vi "Auto Further Switch.vi"(10 "Time to wait (min 50ms)":dbl=100.0, 11 "Right?":bool) -> ()   [LabVIEW 2017]
uses:
  LabVIEW_is_Under_Control.lib/Util/Unpack Gamepad/Button Cluster.ctl
  Team Code/Robot Global Data.vi
panel:
  out "Auto State":T1(ring)
  in  "Time_Limit_ Turn_2":dbl=1500.0 format="%#_13g"
  in  "Time_Limit_fwd_2":dbl=4000.0 format="%#_13g"
  in  "Time_Limit_Turn":dbl=1500.0 format="%#_13g"
  in  "Time_Limit_fwd":dbl=4000.0 format="%#_13g"
  in  "Time_Limit_fwd_3":dbl=1000.0 format="%#_13g"
  in  "Time to wait 3(min 50ms)":dbl=50.0
  in  "Delay Fwd 3":i32=500
  in  "Distance fwd 3":dbl=50.0
  in  "Delay Turn 2":i32=200
  in  "Turn 2":dbl=-90.0 format="%#_13g"
  in  "Delay Fwd 2":i32=200
  in  "Distance fwd 2":dbl=430.0
  in  "Delay Turn":i32=300
  in  "Turn":dbl=-90.0 format="%#_13g"
  in  "Delay Fwd":i32=600
  in  "Distance fwd 1":dbl=600.0
  in  "Time to wait 3 (min 50ms)":dbl=50.0
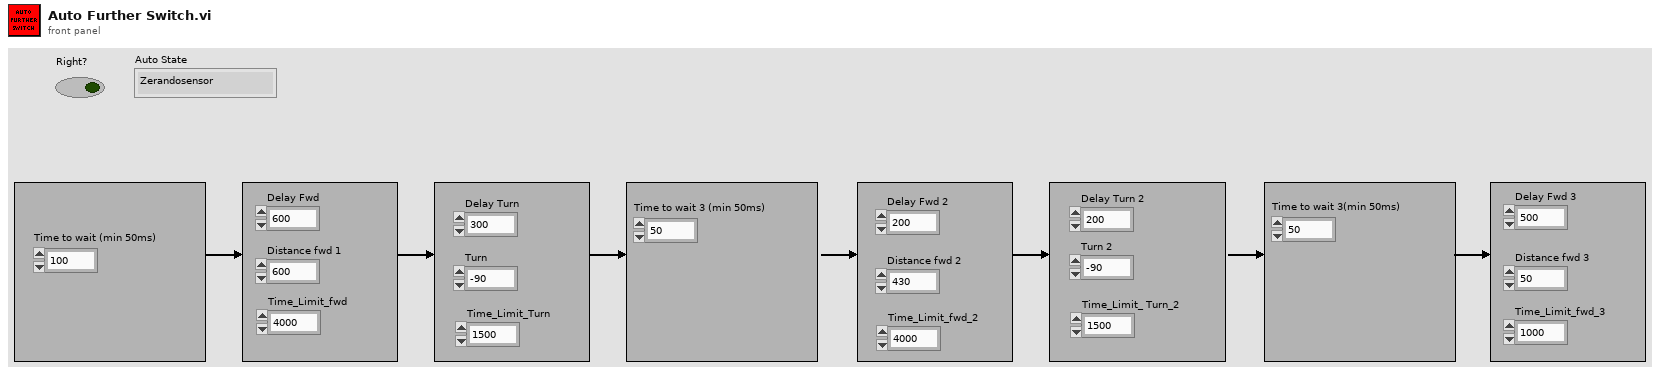
[diagram p1: front panel]
types:
  T1 = enum16{"Zerandosensor", "Andando", "Girando", "Zerandosensor2", "Andando2", "Girando2", "Zerandosensor3", "Andando3", "Score", "Finalizando", "Jogando"}
  T2 = enum16{"Zerandosensor", "Andando", "Girando", "Zerandosensor2", "Andando2", "Girando2", "Zerandosensor3", "Andando3", "Score", "Finalizando"}
  T3 = typedef "Button Cluster.ctl" = cluster{"Buttons[0]":bool, "Buttons[1]":bool, "Buttons[2]":bool, "Buttons[3]":bool, "Buttons[4]":bool, "Buttons[5]":bool, "Buttons[6]":bool, "Buttons[7]":bool, "Buttons[8]":bool, "Buttons[9]":bool}
  T4 = cluster{"proportional gain (Kc)":dbl, "integral time (Ti, min)":dbl, "derivative time (Td, min)":dbl}
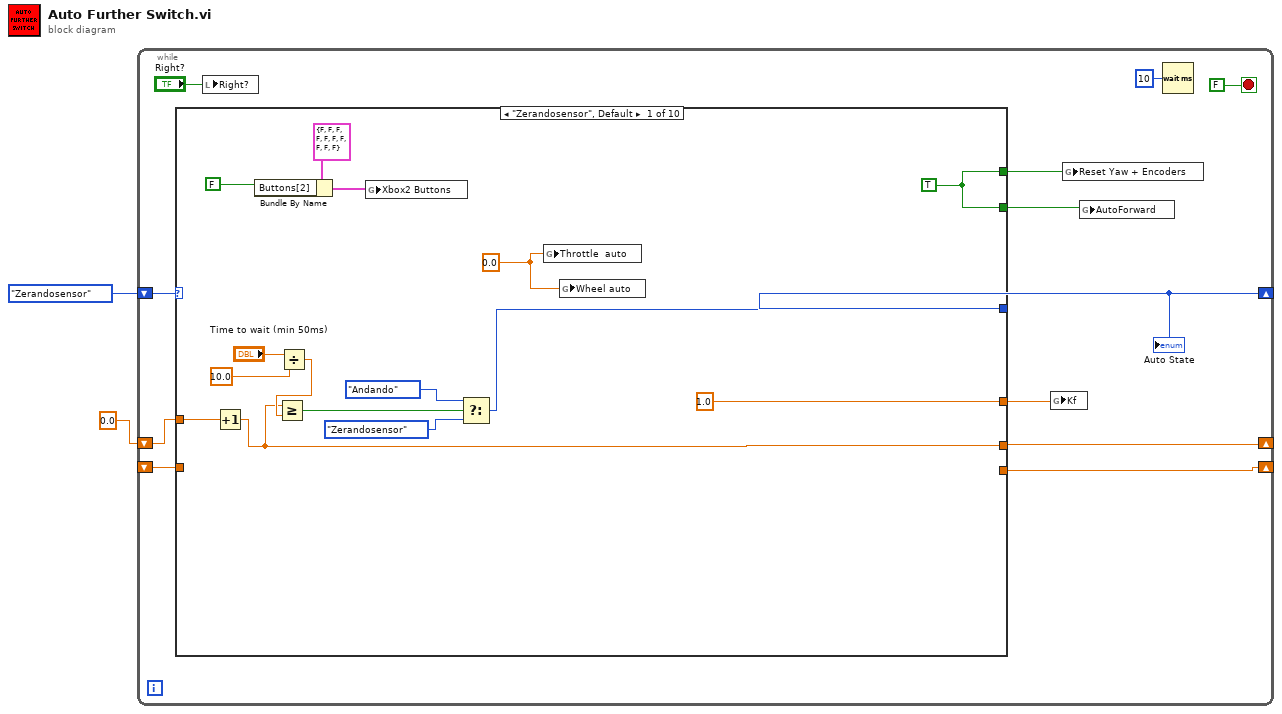
[diagram p0: block diagram]
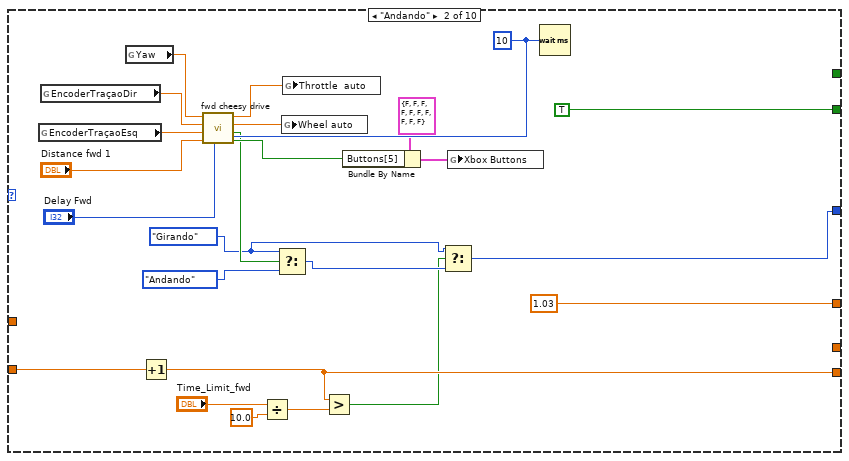
[diagram p2: hidden frame]
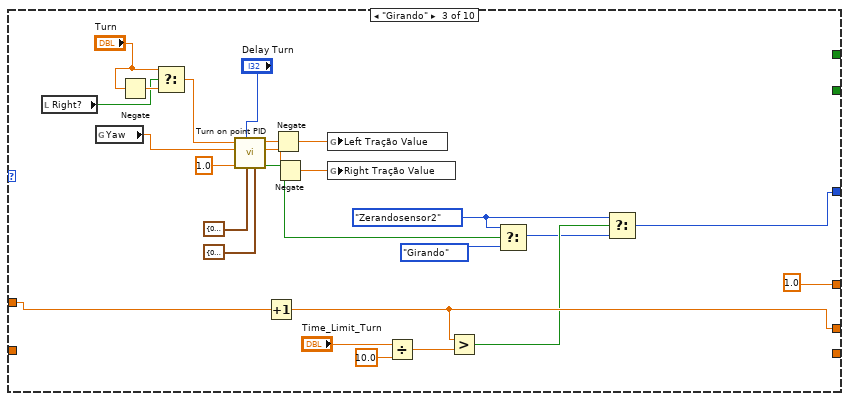
[diagram p3: hidden frame]
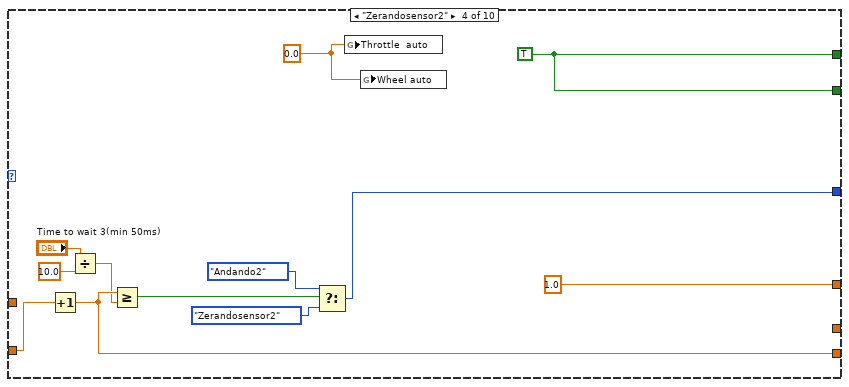
[diagram p4: hidden frame]
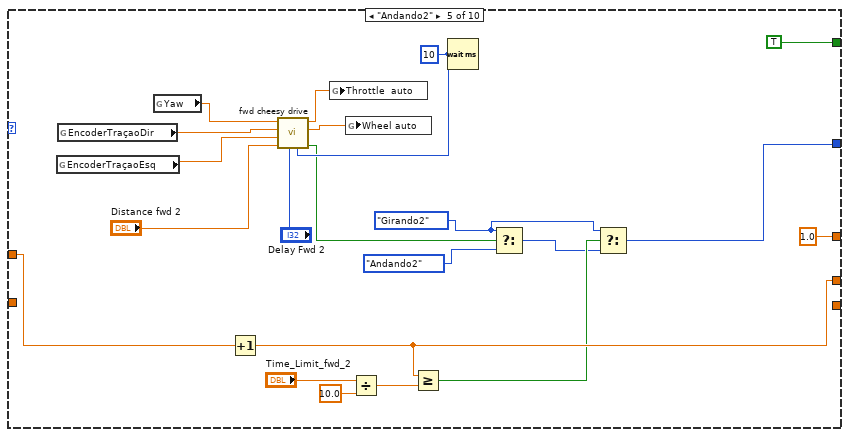
[diagram p5: hidden frame]
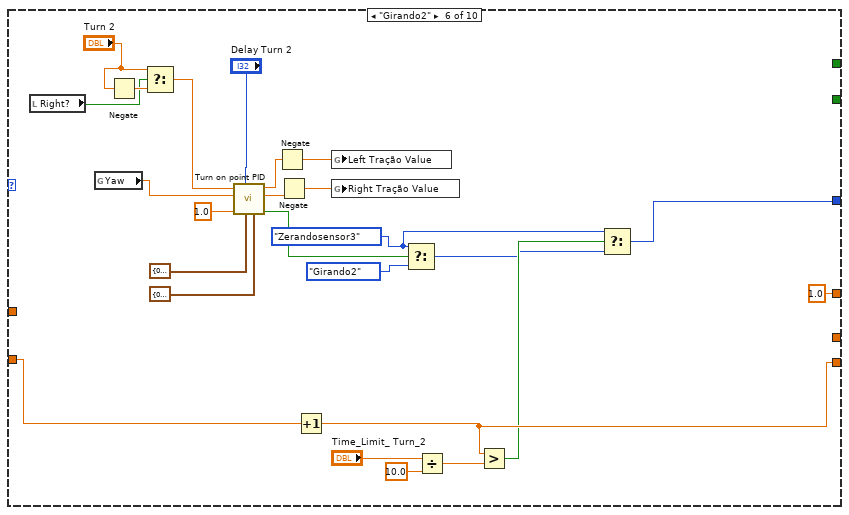
[diagram p6: hidden frame]
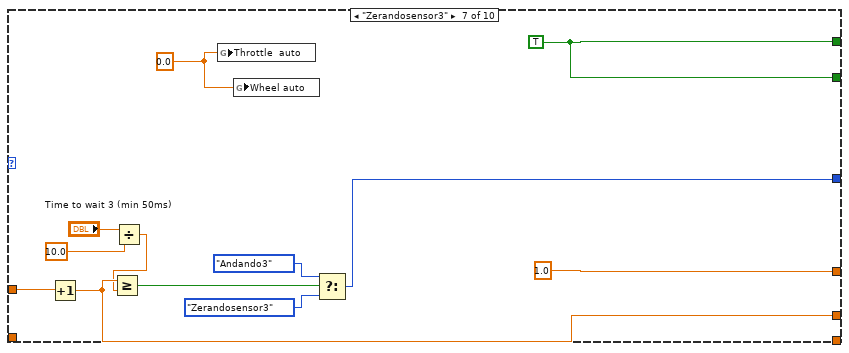
[diagram p7: hidden frame]
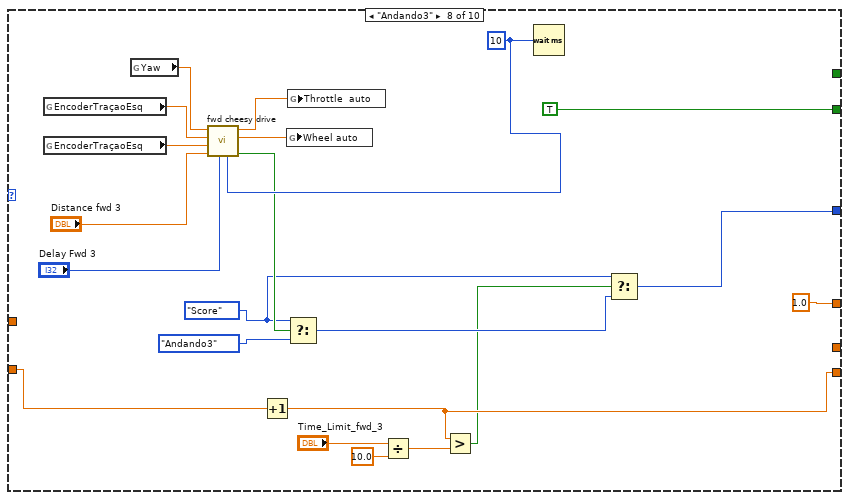
[diagram p8: hidden frame]
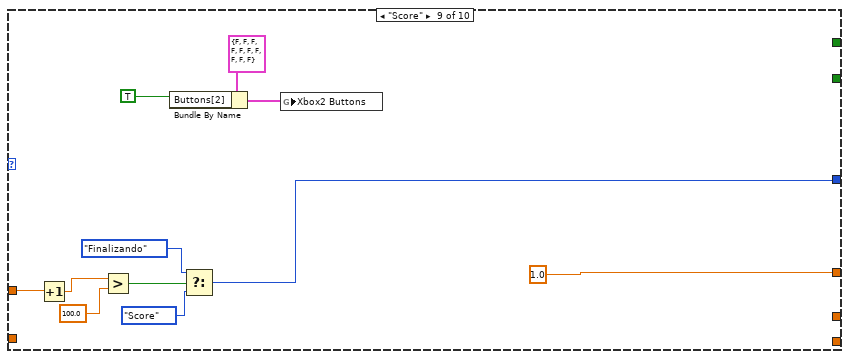
[diagram p9: hidden frame]
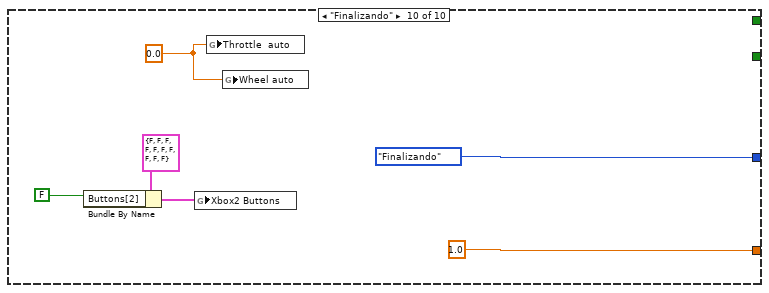
[diagram p10: hidden frame]
diagram:
  n1 = while {
    shift-right: [w6] -> _
    shift-left: T2."Zerandosensor" -> [w5]
    shift-right: [w8] -> _
    shift-left: 0.0 -> [w9]
    shift-right: [w3] -> _
    shift-left: _ -> [w4]
    stop <- FALSE stop-if-true
    n2 = case shown="\"Zerandosensor\", Default" w5 {
      tunnel: [w29 _ _ w88 _ _ w142 _ _ _] -> w11
      tunnel: [w29 TRUE _ w88 TRUE _ w142 TRUE _ _] -> w12
      tunnel: [1.0 1.03 1.0 1.0 1.0 1.0 1.0 1.0 1.0 1.0] -> w10
      tunnel: w9 -> [w25 _ w59 _ w96 _ w146 _ w180 _]
      tunnel: [w15 _ w58 _ w95 _ w138 _ _ _] -> w8
      tunnel: [w22 w34 w57 w86 w91 w116 w141 w153 w173 T1."Finalizando"] -> w6
      tunnel: w4 -> [_ w36 _ w83 _ w118 _ w155 _ _]
      tunnel: [_ w35 _ w82 _ w117 _ w154 _ _] -> w3
      frame "Zerandosensor", Default {
        w23 = 0.0
        w29 = TRUE
        n3 = Increment(x=w25) -> (x+1=w15:dbl)
        n4 = Bundle By Name(cluster=T3 {"Buttons[0]"=FALSE, "Buttons[1]"=FALSE, "Buttons[2]"=FALSE, "Buttons[3]"=FALSE, "Buttons[4]"=FALSE, "Buttons[5]"=FALSE, "Buttons[6]"=FALSE, "Buttons[7]"=FALSE, "Buttons[8]"=FALSE, "Buttons[9]"=FALSE} ("Xbox Buttons"), "Buttons[2]"=FALSE) -> (w18:T3)
        n5 = Divide(x="Time to wait (min 50ms)", y=10.0) -> (x/y=w16:dbl)
        n6 = Greater Or Equal?(x=w15, y=w16) -> (x >= y?=w24:bool)
        n7 = global write "Robot Global Data.vi" "Xbox2 Buttons"(w18) -> ()
        n8 = Select(t=T2."Andando", s=w24, f=T2."Zerandosensor") -> (s? t:f=w22:T2)
        n9 = global write "Robot Global Data.vi" "Throttle  auto"(w23) -> ()
        n10 = global write "Robot Global Data.vi" "Wheel auto"(w23) -> ()
      }
      frame "Andando" {
        w31 = T2."Girando"
        w47 = u32 10 ("milliseconds to wait")
        n11 = global read "Robot Global Data.vi" "EncoderTraçaoEsq"() -> (w50:dbl)
        n12 = global read "Robot Global Data.vi" "EncoderTraçaoDir"() -> (w49:dbl)
        n13 = global read "Robot Global Data.vi" "Yaw"() -> (w51:dbl)
        n14 = Increment(x=w36) -> (x+1=w35:dbl)
        n15 = call "fwd cheesy drive.vi"("Loop Timer"=w47, "Time to stop"="Delay Fwd", "Distance"="Distance fwd 1", "Encoder Left"=w50, "Encoder Right"=w49, "Yaw"=w51) -> ("Finished distance"=w42:bool, "Both finished"=w41:bool, "Direction"=w46:dbl, "Trottle"=w45:dbl)  [unwired: 2 in]
        n16 = Divide(x="Time_Limit_fwd", y=10.0) -> (x/y=w39:dbl)
        n17 = Select(t=w31, s=w41, f=T2."Andando") -> (s? t:f=w32:T2)
        n18 = global write "Robot Global Data.vi" "Wheel auto"(w46) -> ()
        n19 = global write "Robot Global Data.vi" "Throttle  auto"(w45) -> ()
        n20 = Greater?(x=w35, y=w39) -> (0:w30:bool)
        n21 = Bundle By Name(cluster=T3 {"Buttons[0]"=FALSE, "Buttons[1]"=FALSE, "Buttons[2]"=FALSE, "Buttons[3]"=FALSE, "Buttons[4]"=FALSE, "Buttons[5]"=FALSE, "Buttons[6]"=FALSE, "Buttons[7]"=FALSE, "Buttons[8]"=FALSE, "Buttons[9]"=FALSE} ("Xbox Buttons"), "Buttons[5]"=w42) -> (w43:T3)
        n22 = Select(t=w31, s=w30, f=w32) -> (s? t:f=w34:T2)
        n23 = global write "Robot Global Data.vi" "Xbox Buttons"(w43) -> ()
        n24 = Wait (ms)(milliseconds to wait=w47) -> ()  [unwired: 1 out]
      }
      frame "Girando" {
        w54 = T2."Zerandosensor2"
        n25 = local read "Right?"() -> (w66:bool)
        n26 = global read "Robot Global Data.vi" "Yaw"() -> (w72:dbl)
        n27 = Negate(x="Turn") -> (-x=w69:dbl)
        n28 = Select(t="Turn", s=w66, f=w69) -> (s? t:f=w67:dbl)
        n29 = call "Turn on point PID.vi"("Range"=cluster{"output high":dbl, "output low":dbl} {"output high"=0.65, "output low"=-0.65}, "Gains"=T4 {"proportional gain (Kc)"=0.015, "integral time (Ti, min)"=0.01, "derivative time (Td, min)"=0.0}, "Time to stop"="Delay Turn", "Precision"=1.0, "Yaw"=w72, "Setpoint(degrees)"=w67) -> ("Finished?"=w76:bool, "PWM right"=w73:dbl, "PWM left"=w74:dbl)  [unwired: 3 in]
        n30 = Increment(x=w59) -> (x+1=w58:dbl)
        n31 = Negate(x=w74) -> (-x=w71:dbl)
        n32 = Negate(x=w73) -> (-x=w70:dbl)
        n33 = global write "Robot Global Data.vi" "Left Tração Value"(w71) -> ()
        n34 = global write "Robot Global Data.vi" "Right Tração Value"(w70) -> ()
        n35 = Divide(x="Time_Limit_Turn", y=10.0) -> (x/y=w61:dbl)
        n36 = Greater?(x=w58, y=w61) -> (0:w56:bool)
        n37 = Select(t=w54, s=w76, f=T2."Girando") -> (s? t:f=w55:T2)
        n38 = Select(t=w54, s=w56, f=w55) -> (s? t:f=w57:T2)
      }
      frame "Zerandosensor2" {
        w90 = 0.0
        w88 = TRUE
        n39 = Increment(x=w83) -> (x+1=w82:dbl)
        n40 = Divide(x="Time to wait 3(min 50ms)", y=10.0) -> (x/y=w79:dbl)
        n41 = Greater Or Equal?(x=w82, y=w79) -> (x >= y?=w87:bool)
        n42 = Select(t=T2."Andando2", s=w87, f=T2."Zerandosensor2") -> (s? t:f=w86:T2)
        n43 = global write "Robot Global Data.vi" "Throttle  auto"(w90) -> ()
        n44 = global write "Robot Global Data.vi" "Wheel auto"(w90) -> ()
      }
      frame "Andando2" {
        w92 = T2."Girando2"
        w105 = u32 10 ("milliseconds to wait")
        n45 = global read "Robot Global Data.vi" "EncoderTraçaoEsq"() -> (w108:dbl)
        n46 = global read "Robot Global Data.vi" "EncoderTraçaoDir"() -> (w107:dbl)
        n47 = global read "Robot Global Data.vi" "Yaw"() -> (w109:dbl)
        n48 = Increment(x=w96) -> (x+1=w95:dbl)
        n49 = call "fwd cheesy drive.vi"("Loop Timer"=w105, "Time to stop"="Delay Fwd 2", "Distance"="Distance fwd 2", "Encoder Left"=w108, "Encoder Right"=w107, "Yaw"=w109) -> ("Finished distance"=w100:bool, "Direction"=w103:dbl, "Trottle"=w102:dbl)  [unwired: 2 in, 1 out]
        n50 = global write "Robot Global Data.vi" "Throttle  auto"(w102) -> ()
        n51 = global write "Robot Global Data.vi" "Wheel auto"(w103) -> ()
        n52 = Divide(x="Time_Limit_fwd_2", y=10.0) -> (x/y=w98:dbl)
        n53 = Greater Or Equal?(x=w95, y=w98) -> (x >= y?=w94:bool)
        n54 = Wait (ms)(milliseconds to wait=w105) -> ()  [unwired: 1 out]
        n55 = Select(t=w92, s=w100, f=T2."Andando2") -> (s? t:f=w93:T2)
        n56 = Select(t=w92, s=w94, f=w93) -> (s? t:f=w91:T2)
      }
      frame "Girando2" {
        w115 = T2."Zerandosensor3"
        n57 = local read "Right?"() -> (w124:bool)
        n58 = global read "Robot Global Data.vi" "Yaw"() -> (w130:dbl)
        n59 = Negate(x="Turn 2") -> (-x=w127:dbl)
        n60 = Select(t="Turn 2", s=w124, f=w127) -> (s? t:f=w125:dbl)
        n61 = call "Turn on point PID.vi"("Range"=cluster{"output high":dbl, "output low":dbl} {"output high"=0.65, "output low"=-0.65}, "Gains"=T4 {"proportional gain (Kc)"=0.015, "integral time (Ti, min)"=0.01, "derivative time (Td, min)"=0.0}, "Time to stop"="Delay Turn 2", "Precision"=1.0, "Yaw"=w130, "Setpoint(degrees)"=w125) -> ("Finished?"=w134:bool, "PWM right"=w131:dbl, "PWM left"=w132:dbl)  [unwired: 3 in]
        n62 = Negate(x=w132) -> (-x=w129:dbl)
        n63 = Negate(x=w131) -> (-x=w128:dbl)
        n64 = Increment(x=w118) -> (x+1=w117:dbl)
        n65 = global write "Robot Global Data.vi" "Left Tração Value"(w129) -> ()
        n66 = global write "Robot Global Data.vi" "Right Tração Value"(w128) -> ()
        n67 = Select(t=w115, s=w134, f=T2."Girando2") -> (s? t:f=w112:T2)
        n68 = Divide(x="Time_Limit_ Turn_2", y=10.0) -> (x/y=w120:dbl)
        n69 = Greater?(x=w117, y=w120) -> (0:w113:bool)
        n70 = Select(t=w115, s=w113, f=w112) -> (s? t:f=w116:T2)
      }
      frame "Zerandosensor3" {
        w142 = TRUE
        w144 = 0.0
        n71 = Increment(x=w146) -> (x+1=w138:dbl)
        n72 = Divide(x="Time to wait 3 (min 50ms)", y=10.0) -> (x/y=w137:dbl)
        n73 = Greater Or Equal?(x=w138, y=w137) -> (x >= y?=w145:bool)
        n74 = global write "Robot Global Data.vi" "Throttle  auto"(w144) -> ()
        n75 = global write "Robot Global Data.vi" "Wheel auto"(w144) -> ()
        n76 = Select(t=T2."Andando3", s=w145, f=T2."Zerandosensor3") -> (s? t:f=w141:T2)
      }
      frame "Andando3" {
        w151 = T2."Score"
        w160 = u32 10 ("milliseconds to wait")
        n77 = global read "Robot Global Data.vi" "EncoderTraçaoEsq"() -> (w165:dbl)
        n78 = global read "Robot Global Data.vi" "EncoderTraçaoEsq"() -> (w166:dbl)
        n79 = global read "Robot Global Data.vi" "Yaw"() -> (w167:dbl)
        n80 = call "fwd cheesy drive.vi"("Loop Timer"=w160, "Time to stop"="Delay Fwd 3", "Distance"="Distance fwd 3", "Encoder Left"=w166, "Encoder Right"=w165, "Yaw"=w167) -> ("Finished distance"=w159:bool, "Direction"=w162:dbl, "Trottle"=w161:dbl)  [unwired: 2 in, 1 out]
        n81 = Increment(x=w155) -> (x+1=w154:dbl)
        n82 = global write "Robot Global Data.vi" "Wheel auto"(w162) -> ()
        n83 = global write "Robot Global Data.vi" "Throttle  auto"(w161) -> ()
        n84 = Select(t=w151, s=w159, f=T2."Andando3") -> (s? t:f=w150:T2)
        n85 = Divide(x="Time_Limit_fwd_3", y=10.0) -> (x/y=w158:dbl)
        n86 = Greater?(x=w154, y=w158) -> (0:w149:bool)
        n87 = Wait (ms)(milliseconds to wait=w160) -> ()  [unwired: 1 out]
        n88 = Select(t=w151, s=w149, f=w150) -> (s? t:f=w153:T2)
      }
      frame "Score" {
        n89 = Increment(x=w180) -> (x+1=w179:dbl)
        n90 = Greater?(x=w179, y=100.0) -> (0:w177:bool)
        n91 = Bundle By Name(cluster=T3 {"Buttons[0]"=FALSE, "Buttons[1]"=FALSE, "Buttons[2]"=FALSE, "Buttons[3]"=FALSE, "Buttons[4]"=FALSE, "Buttons[5]"=FALSE, "Buttons[6]"=FALSE, "Buttons[7]"=FALSE, "Buttons[8]"=FALSE, "Buttons[9]"=FALSE} ("Xbox Buttons"), "Buttons[2]"=TRUE) -> (w171:T3)
        n92 = Select(t=T1."Finalizando", s=w177, f=T1."Score") -> (s? t:f=w173:T1)
        n93 = global write "Robot Global Data.vi" "Xbox2 Buttons"(w171) -> ()
      }
      frame "Finalizando" {
        w186 = 0.0
        n94 = Bundle By Name(cluster=T3 {"Buttons[0]"=FALSE, "Buttons[1]"=FALSE, "Buttons[2]"=FALSE, "Buttons[3]"=FALSE, "Buttons[4]"=FALSE, "Buttons[5]"=FALSE, "Buttons[6]"=FALSE, "Buttons[7]"=FALSE, "Buttons[8]"=FALSE, "Buttons[9]"=FALSE} ("Xbox Buttons"), "Buttons[2]"=FALSE) -> (w182:T3)
        n95 = global write "Robot Global Data.vi" "Xbox2 Buttons"(w182) -> ()
        n96 = global write "Robot Global Data.vi" "Throttle  auto"(w186) -> ()
        n97 = global write "Robot Global Data.vi" "Wheel auto"(w186) -> ()
      }
    }
    "Auto State" <- w6
    n98 = local write "Right?"("Right?") -> ()
    n99 = global write "Robot Global Data.vi" "Kf"(w10) -> ()
    n100 = global write "Robot Global Data.vi" "Reset Yaw + Encoders"(w11) -> ()
    n101 = global write "Robot Global Data.vi" "AutoForward"(w12) -> ()
    n102 = Wait (ms)(milliseconds to wait=u32 10) -> ()  [unwired: 1 out]
  }
